vi "插件_均匀白噪声.vi"() -> ()   [LabVIEW 2013]
uses:
  <vilib>/measure/NI_MABase.lvlib
panel:
  in  "停止":bool
  out "波形图":waveform(dbl)(graph)
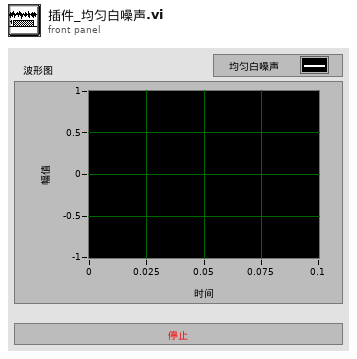
[diagram p1: front panel]
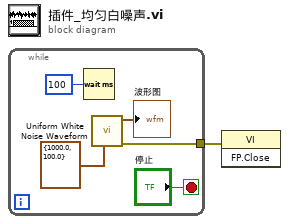
[diagram p0: block diagram]
diagram:
  n1 = while {
    tunnel: [w2] -> w1
    stop <- "停止" stop-if-true
    n2 = Wait (ms)(milliseconds to wait=u32 100 ("等待时间（毫秒）")) -> ()  [unwired: 1 out]
    n3 = call <vilib>:"Uniform White Noise Waveform.vi"("sampling info"=cluster{"Fs":dbl, "#s":dbl} {"Fs"=1000.0, "#s"=100.0}) -> ("error out"=w2:errorcluster, "signal out"=→"波形图":waveform(dbl))  [unwired: 9 in]
  }
  n4 = invoke class="VI" method="FP.Close"(error in=w1) -> ()  [unwired: 2 in, 3 out]
